vi "Get Numeric Value.vi"(8 "error in (no error)":errorcluster, 11 "Ctl Ref":refnum<vi>) -> (0 "error out":errorcluster, 3 "Numeric Value":dbl)   [LabVIEW 2020, in "MacroAssert.lvlib" / "Numeric Assertion.lvclass"]
uses:
  Numeric Assertion.lvclass
  Numeric Assertion.lvclass/Numeric Assertion.ctl
  MacroAssert.lvlib
  SubVIs/Custom Errors/Custom Errors.lvlib
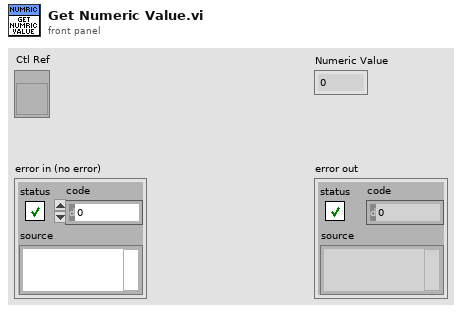
[diagram p1: front panel]
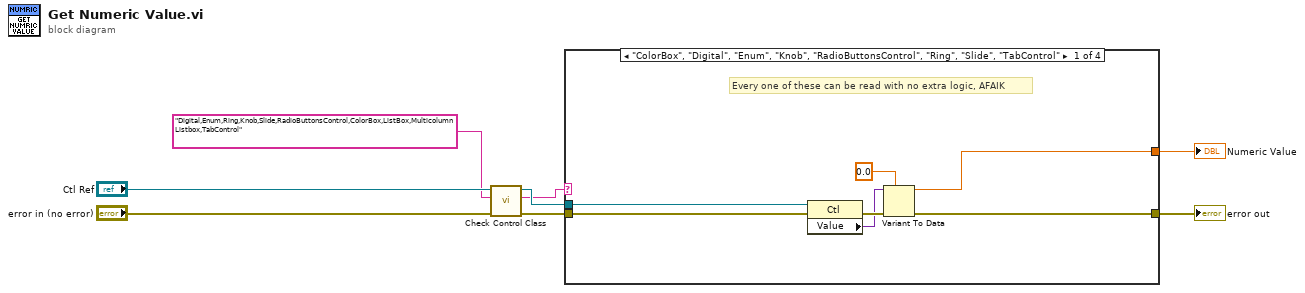
[diagram p0: block diagram]
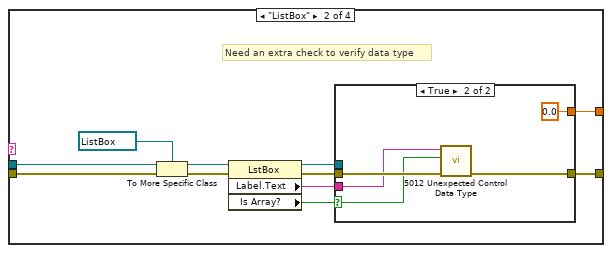
[diagram p2: hidden frame]
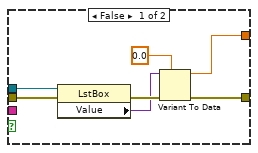
[diagram p3: hidden frame]
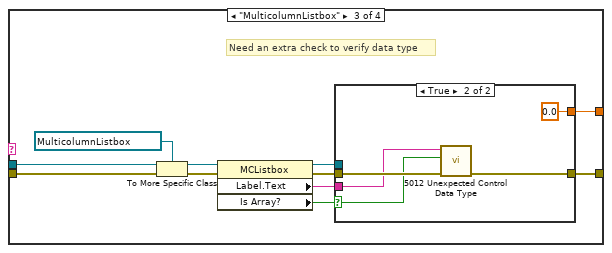
[diagram p4: hidden frame]
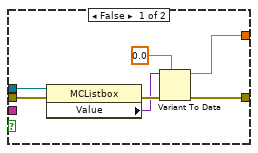
[diagram p5: hidden frame]
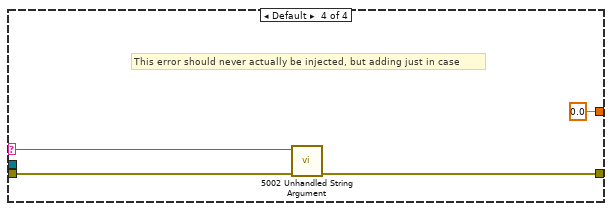
[diagram p6: hidden frame]
diagram:
  n1 = call "Check Control Class.vi"("error in (no error)"="error in (no error)", "Supported Classes"="Digital,Enum,Ring,Knob,Slide,RadioButtonsControl,ColorBox,ListBox,MulticolumnListbox,TabControl", "Ctl Ref"="Ctl Ref") -> ("error out"=w3:errorcluster, "Class Name"=w1:string, "Ctl Ref out"=w2:refnum<vi>)  [unwired: 6 in]
  n2 = case shown="\"ColorBox\", \"Digital\", \"Enum\", \"Knob\", \"RadioButtonsControl\", \"Ring\", \"Slide\", \"TabControl\"" w1 {
    selector: w1 -> [_ _ _ w62]
    tunnel: w3 -> [w15 w26 w49 w65]
    tunnel: [w14 w19 w42 w64] -> w8
    tunnel: w2 -> [w12 w24 w47 _]
    tunnel: [w9 w18 w41 0.0] -> w4
    frame "ColorBox", "Digital", "Enum", "Knob", "RadioButtonsControl", "Ring", "Slide", "TabControl" {
      # "Every one of these can be read with no extra logic, AFAIK"
      n3 = property class="Ctl"(reference=w12, error in=w15) -> (error out=w13:errorcluster, "Value"=w10:variant)  [unwired: 1 out]
      n4 = Variant To Data(error in=w13, type=0.0, Variant=w10) -> (data=w9:dbl, error out=w14:errorcluster)
    }
    frame "ListBox" {
      # "Need an extra check to verify data type"
      n5 = To More Specific Class(target class=refnum<vi> refnum ("reference out"), reference=w24, error in=w26) -> (specific class reference=w22:refnum<vi>, error out=w23:errorcluster)
      n6 = property class="LstBox"(reference=w22, error in=w23) -> (reference out=w20:refnum<vi>, error out=w21:errorcluster, "Label.Text"=w16:string, "Is Array?"=w17:bool)
      n7 = case shown="True" w17 {
        selector: w17 -> [_ w35]
        tunnel: w21 -> [w30 w38]
        tunnel: w20 -> [w29 _]
        tunnel: [w28 w37] -> w19
        tunnel: [w27 0.0] -> w18
        tunnel: w16 -> [_ w36]
        frame False {
          n8 = property class="LstBox"(reference=w29, error in=w30) -> (error out=w33:errorcluster, "Value"=w31:variant)  [unwired: 1 out]
          n9 = Variant To Data(error in=w33, type=0.0, Variant=w31) -> (data=w27:dbl, error out=w28:errorcluster)
        }
        frame True {
          n10 = call "5012 Unexpected Control Data Type.vi"("error in (no error)"=w38, "Expecting Scalar?"=w35, "Control Name"=w36) -> ("error out"=w37:errorcluster)  [unwired: 8 in]
        }
      }
    }
    frame "MulticolumnListbox" {
      # "Need an extra check to verify data type"
      n11 = To More Specific Class(target class=refnum<vi> refnum ("reference out"), reference=w47, error in=w49) -> (specific class reference=w45:refnum<vi>, error out=w46:errorcluster)
      n12 = property class="MCListbox"(reference=w45, error in=w46) -> (reference out=w43:refnum<vi>, error out=w44:errorcluster, "Label.Text"=w39:string, "Is Array?"=w40:bool)
      n13 = case shown="True" w40 {
        selector: w40 -> [_ w58]
        tunnel: w44 -> [w53 w61]
        tunnel: w43 -> [w52 _]
        tunnel: [w51 w60] -> w42
        tunnel: [w50 0.0] -> w41
        tunnel: w39 -> [_ w59]
        frame False {
          n14 = property class="MCListbox"(reference=w52, error in=w53) -> (error out=w56:errorcluster, "Value"=w54:variant)  [unwired: 1 out]
          n15 = Variant To Data(error in=w56, type=0.0, Variant=w54) -> (data=w50:dbl, error out=w51:errorcluster)
        }
        frame True {
          n16 = call "5012 Unexpected Control Data Type.vi"("error in (no error)"=w61, "Expecting Scalar?"=w58, "Control Name"=w59) -> ("error out"=w60:errorcluster)  [unwired: 8 in]
        }
      }
    }
    frame Default {
      # "This error should never actually be injected, but adding just in case"
      n17 = call "5002 Unhandled String Argument.vi"("error in (no error)"=w65, "Argument"=w62) -> ("error out"=w64:errorcluster)  [unwired: 9 in]
    }
  }
  "error out" <- w8
  "Numeric Value" <- w4
